vi "Recode by Column.vi"(10 "Input Subtable":string[][](array[string]), 11 "Column Headers":string[](array[string])) -> (2 "Output Subtable":string[][](array[string]))   [LabVIEW 2010]
panel:
  in  "Cancel":bool
  in  "Accept":bool
  in  "New Values":string[](array[string])
  out "Old Values":string[](array[string])
  in  "Column to recode":u16(ring) items=["Unique_ID", "LayerID", "Sample_Name", "Date-Time", "User_Name", "Filename", "File_Date-Time", "Temperature(K)", "Current(A)", "Delay(Sec)", "Distance(um)", "Magnetic_Field_Strength(T)", "Notes", "Bulk_Concentration(cm-3)", "Mobility(cm2/Vs)", "Resistivity(ohm*cm)", "Magneto-Resistance", "Sheet_Concentration(cm-2)", "Avg_Hall_Coefficient", "Conductivity(G/cm)", "Data_Verified", "Symmetry_Test", "Symmetry_Test_(%)", "Voltage_Test", "Voltage_Test_(%)", "Cross-Hall_Test", "Cross-Hall_(%)"]
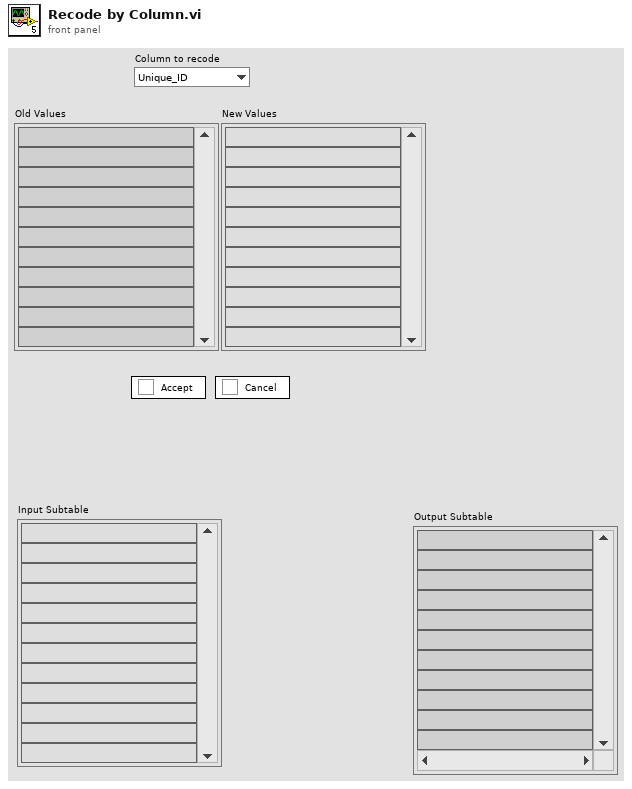
[diagram p1: front panel]
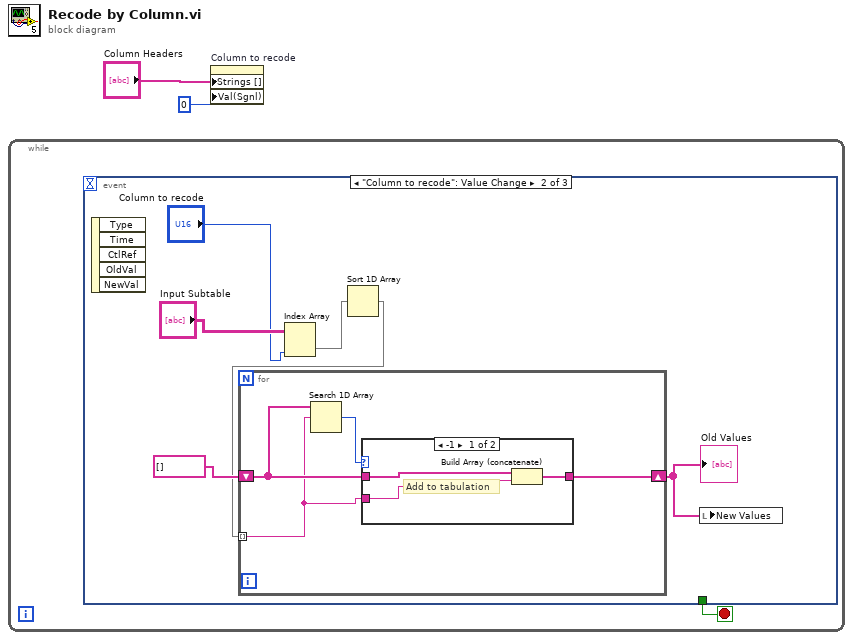
[diagram p0: block diagram]
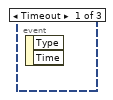
[diagram p2: hidden frame]
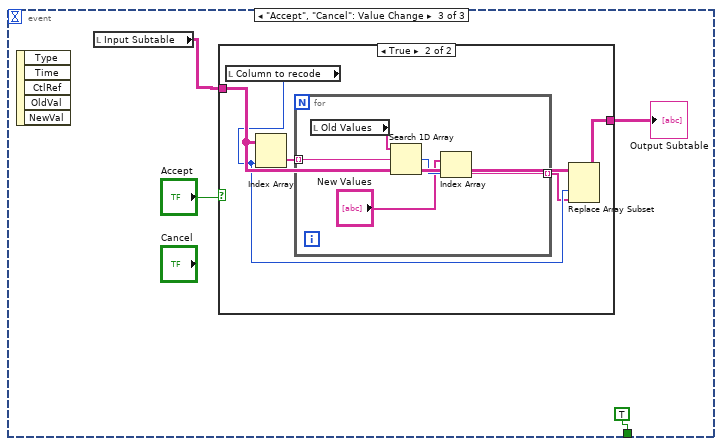
[diagram p4: hidden frame]
diagram:
  n1 = while {
    stop <- w3 stop-if-true
    n2 = event shown="[1] \"Column to recode\": Value Change" {
      selector: _ -> [_ _ _]
      dyn-events: _ -> [_ _ _]
      timeout: _ -> [_ _ _]
      tunnel: [_ _ TRUE] -> w3
      event Timeout {
        n3 = event-data() -> ()  [unwired: 1 in, 2 out]
      }
      event "Column to recode": Value Change {
        n4 = event-data() -> ()  [unwired: 1 in, 5 out]
        n5 = Index Array(array="Input Subtable", index (col)="Column to recode") -> (element=w8:string[])  [unwired: 1 in]
        n6 = Sort 1D Array(array=w8) -> (sorted array=w6:string[])
        n7 = for {
          tunnel: w6 -> [w11] mode=indexing
          shift-right: [w13] -> w5
          shift-left: string[] [] -> [w12]
          n8 = Search 1D Array(1D array=w12, element=w11) -> (index of element=w10:i32)  [unwired: 1 in]
          n9 = case shown="-1" w10 {
            tunnel: w11 -> [w16 _]
            tunnel: [w15 w17] -> w13
            tunnel: w12 -> [w14 w17]
            frame -1 {
              # "Add to tabulation"
              n10 = Build Array (concatenate)(w14, w16) -> (w15:string[])
            }
            frame Default {
              # "Don't Add"
            }
          }
        }
        "Old Values" <- w5
        n11 = local write "New Values"(w5) -> ()
      }
      event "Accept", "Cancel": Value Change {
        n12 = event-data() -> ()  [unwired: 1 in, 5 out]
        n13 = local read "Input Subtable"() -> (w19:string[][])
        n14 = case shown="True" "Accept" {
          tunnel: w19 -> [w22 w26]
          tunnel: [w22 w23] -> w18
          frame False {
          }
          frame True {
            n15 = local read "Column to recode"() -> (w25:u16)
            n16 = Index Array(array=w26, index (col)=w25) -> (element=w27:string[])  [unwired: 1 in]
            n17 = for {
              tunnel: w27 -> [w32] mode=indexing
              tunnel: [w28] -> w24 mode=indexing
              n18 = local read "Old Values"() -> (w31:string[])
              n19 = Search 1D Array(1D array=w31, element=w32) -> (index of element=w30:i32)  [unwired: 1 in]
              n20 = Index Array(array="New Values", index=w30) -> (element=w28:string)
            }
            n21 = Replace Array Subset(array=w26, new element=w24, index (col)=w25) -> (w23:string[][])  [unwired: 1 in]
          }
        }
        "Output Subtable" <- w18
      }
    }
  }
  n22 = property on="Column to recode" class="Ring (strict)"("Strings []"="Column Headers", "Val(Sgnl)"=u16 0 ("Value (Signaling)")) -> ()  [unwired: 2 in, 2 out]
